vi "TGA_Configuration.vi"() -> ()   [LabVIEW 2016]
uses:
  TGA_Furnace_v230504.llb/LogInterval.ctl
  TGA_Furnace_v230504.llb/ChartWidth.ctl
  TGA_Furnace_v230504.llb/ADAM_models_enu.ctl
  TGA_Furnace_v230504.llb/Config_cluster.ctl
  TGA_Furnace_v230504.llb/HW_Config_cluster.ctl
  TGA_Furnace_v230504.llb/Adam_ID_cluster.ctl
  TGA_Furnace_v230504.llb/MFCs_ID_cluster.ctl
  TGA_Furnace_v230504.llb/MFC_ID_cluster.ctl
panel:
  in  "Gas Setpoints 3":T1={"Flow SP (l/min)"=15.0, "F1 N2 (%)"=79.99999999999997, "F1 H2 (%)"=0.0, "F1 CO (%)"=0.0, "F1 CO2 (%)"=20.00000000000003} caption="Gas Setpoints" {"F1 H2 (%)" min=0.0 max=100.0 step=0.1 format="%.1f"; "F1 CO2 (%)" min=0.0 max=100.0 step=0.1 format="%.1f"; "F1 CO (%)" min=0.0 max=100.0 step=0.1 format="%.1f"; "F1 N2 (%)" min=-10.0 max=100.0 format="%.1f"; "Flow SP (l/min)" min=0.0 max=30.0 format="%.1f"}
  in  "Gas Setpoints 2":T1={"Flow SP (l/min)"=15.0, "F1 N2 (%)"=79.99999999999997, "F1 H2 (%)"=0.0, "F1 CO (%)"=0.0, "F1 CO2 (%)"=20.00000000000003} caption="Gas Setpoints" {"F1 H2 (%)" min=0.0 max=100.0 step=0.1 format="%.1f"; "F1 CO2 (%)" min=0.0 max=100.0 step=0.1 format="%.1f"; "F1 CO (%)" min=0.0 max=100.0 step=0.1 format="%.1f"; "F1 N2 (%)" min=-10.0 max=100.0 format="%.1f"; "Flow SP (l/min)" min=0.0 max=30.0 format="%.1f"}
  in  "Gas Setpoints":T1={"Flow SP (l/min)"=15.0, "F1 N2 (%)"=79.99999999999997, "F1 H2 (%)"=0.0, "F1 CO (%)"=0.0, "F1 CO2 (%)"=20.00000000000003} {"F1 H2 (%)" min=0.0 max=100.0 step=0.1 format="%.1f"; "F1 CO2 (%)" min=0.0 max=100.0 step=0.1 format="%.1f"; "F1 CO (%)" min=0.0 max=100.0 step=0.1 format="%.1f"; "F1 N2 (%)" min=-10.0 max=100.0 format="%.1f"; "Flow SP (l/min)" min=0.0 max=30.0 format="%.1f"}
  out "Changed":bool
  in  "SaveAs_btn":bool
  in  "cancel_btn":bool
  in  "save_btn":bool
  in  "Tab Control":T2(tab)
  in  "Data directory path":path=path "C:/TGA/Data"
  in  "LogInterval":T3=1 items=["1 second"=1, "2 seconds"=2, "5 seconds"=5, "10 seconds"=10, "20 seconds"=20, "30 seconds"=30, "1 minute"=60, "2 minutes"=120, "5 minutes"=300]
  in  "LogStartComment":bool caption="Allow comment at start of logging."
  in  "LogEndComment":bool caption="Allow comment at end of logging"
  in  "GraphWidth":T4=1 items=["1 Minute", "5 Minutes", "10 Minutes", "30 Minutes", "1 Hour", "2 Hours"]
  in  "GraphSizeLimit":u16=7200
  in  "AlarmDelay":dbl=30.0 caption="N2 Flow Alarm\nDelay (s)"
  in  "Flow_error%":dbl=20.0 caption="N2 Low Flow\nError (%)"
  in  "TGA Gas File":string="Default" caption="Gas Filename"
  in  "Gas_SPs":T5={"Flow SP"=15.0, "N2 (%)"=70.0, "H2 (%)"=0.0, "CO (%)"=10.0, "CO2 (%)"=20.0} {"H2 (%)" min=0.0 max=100.0 format="%.1f"; "CO2 (%)" min=0.0 max=100.0 format="%.1f"; "CO (%)" min=0.0 max=100.0 format="%.1f"; "N2 (%)" min=-10.0 max=100.0 format="%.1f"; "Flow SP" min=0.0 max=30.0 format="%.1f"}
  out "ConfigFile path":path=path "C:/TGA/TGA_Main_v220630.cfg"
  out "MFCs_found":T6
  out "Adam_out_found":bool caption="Adam 4050"
  out "Euro_found":bool caption="Eurotherm"
  out "Balance_found":bool caption="Balance"
  in  "Adam_Out_ID":T8={"Serial Port"="COM7", "Model"=enum."4050", "Address"=1, "Slot"=0} caption="Adam Gas Solenoid\nOutput Module" {"Slot" max=7; "Address" min=1 max=254}
  in  "Euro_Address":u8=1 min=1 max=254
  in  "Euro_Port":refnum<visa-resource-name>="COM5" caption="Eurothem Temp.\nController Port"
  in  "Adam_In_ID":T8={"Serial Port"="COM6", "Model"=enum."4017", "Address"=2, "Slot"=0} caption="Adam Temp.\nInput Module" {"Slot" max=7; "Address" min=1 max=254}
  in  "Balance_Port":refnum<visa-resource-name>="COM4" caption="Radwag Balance\nSerial Port"
  in  "MFCs_Port":refnum<visa-resource-name>="COM10" caption="Brooks Mass Flow\nControllers Port"
  in  "test_btns":T9
  out "Adam_in_found":bool caption="Adam 4018"
  in  "MFC Device IDs":T10={"F1N2 MFC Device ID"={"MFC Device ID"=751101, "Type"=50}, "F1H2 MFC Device ID"={"MFC Device ID"=98201001, "Type"=100}, "F1CO MFC Device ID"={"MFC Device ID"=751201, "Type"=50}, "F1CO2 MFC Device ID"={"MFC Device ID"=98202001, "Type"=100}}
  # "TGA Configuration Editor"
  # "Type"
  # "Type"
  # "Type"
  # "Type"
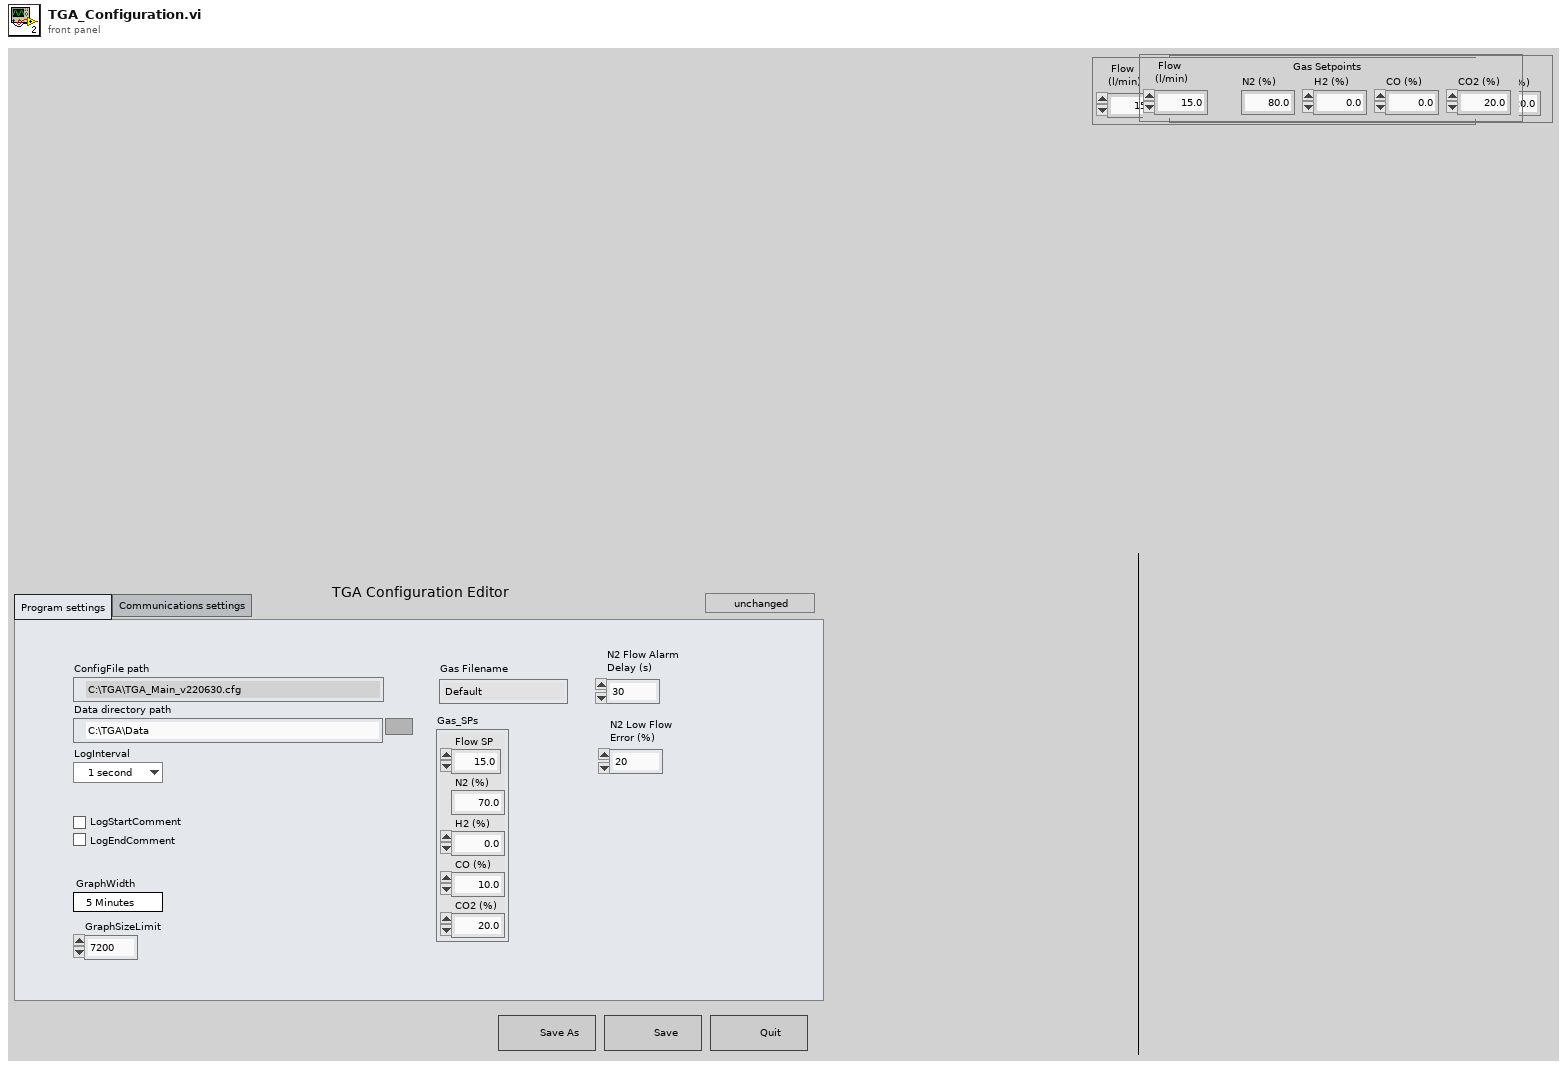
[diagram p1: front panel]
types:
  T1 = cluster{"Flow SP (l/min)":dbl, "F1 N2 (%)":dbl, "F1 H2 (%)":dbl, "F1 CO (%)":dbl, "F1 CO2 (%)":dbl}
  T2 = enum32{"Program settings", "Communications settings"}
  T3 = typedef "LogInterval.ctl" = u16
  T4 = typedef "ChartWidth.ctl" = u16
  T5 = cluster{"Flow SP":dbl, "N2 (%)":dbl, "H2 (%)":dbl, "CO (%)":dbl, "CO2 (%)":dbl}
  T6 = cluster{"Adam_out_found":bool, "Adam_out_found 2":bool, "Adam_out_found 3":bool, "Adam_out_found 4":bool}
  T7 = typedef "ADAM_models_enu.ctl" = enum16{"4011", "4012", "4013", "4015", "4015T", "4016", "4017", "4017+", "4018", "4018+", "4019+", "4019M", "4021", "4024", "4050", "4051", "4052", "4053", "4055", "4056S", "4056SO", "4060", "4068", "4069", "5000", "5017", "5018", "5024", "5051"}
  T8 = cluster{"Serial Port":refnum<visa-resource-name>, "Model":T7, "Address":u8, "Slot":u8}
  T9 = cluster{"test_bal_btn":bool, "test_adam_in":bool, "test_euro_btn":bool, "test_adam_out":bool, "test_MFCs_btn":bool}
  T10 = cluster{"F1N2 MFC Device ID":cluster{"MFC Device ID":u32, "Type":u8}, "F1H2 MFC Device ID":cluster{"MFC Device ID":u32, "Type":u8}, "F1CO MFC Device ID":cluster{"MFC Device ID":u32, "Type":u8}, "F1CO2 MFC Device ID":cluster{"MFC Device ID":u32, "Type":u8}}
  T11 = enum32{"Invalid", "Standard", "Closed", "Hidden", "Minimized", "Maximized"}
  T12 = typedef "Config_cluster.ctl" = cluster{"ConfigFile path":path, "Data directory path":path, "LogInterval":T3, "LogStartComment":bool, "LogEndComment":bool, "GraphWidth":T4, "GraphSizeLimit":u16, "HW_Config_cluster":T13, "TGA Gas File":string, "Gas_SPs":cluster{"Flow SP":dbl, "N2 (%)":dbl, "H2 (%)":dbl, "CO (%)":dbl, "CO2 (%)":dbl}, "AlarmDelay":dbl, "Flow_error%":dbl, "Purge Flow":dbl, "Gas_Times":cluster{"PrePurge Time":dbl, "Reduction Time":dbl, "Purge Time":dbl}, "Purge Setpoints":cluster{"F1 N2 (%)":dbl, "F1 H2 (%)":dbl, "F1 CO (%)":dbl, "F1 CO2 (%)":dbl}}
  T13 = typedef "HW_Config_cluster.ctl" = cluster{"Balance_Port":refnum<visa-resource-name>, "Adam_In_ID":T14, "Euro_Port":refnum<visa-resource-name>, "Euro_Address":u8, "Adam_Out_ID":T14, "MFCs_Port":refnum<visa-resource-name>, "MFC Device IDs":T15}
  T14 = typedef "Adam_ID_cluster.ctl" = cluster{"Serial Port":refnum<visa-resource-name>, "Model":T7, "Address":u8, "Slot":u8}
  T15 = typedef "MFCs_ID_cluster.ctl" = cluster{"F1N2 MFC Device ID":T16, "F1H2 MFC Device ID":T16, "F1CO MFC Device ID":T16, "F1CO2 MFC Device ID":T16}
  T16 = typedef "MFC_ID_cluster.ctl" = cluster{"MFC Device ID":u32, "Type":u8}
  T17 = cluster{"ConfigFile path":bool, "Data directory path":bool, "LogInterval":bool, "LogStartComment":bool, "LogEndComment":bool, "GraphWidth":bool, "GraphSizeLimit":bool, "HW_Config_cluster":cluster{"Balance_Port":bool, "Adam_In_ID":cluster{"Serial Port":bool, "Model":bool, "Address":bool, "Slot":bool}, "Euro_Port":bool, "Euro_Address":bool, "Adam_Out_ID":cluster{"Serial Port":bool, "Model":bool, "Address":bool, "Slot":bool}, "MFCs_Port":bool, "MFC Device IDs":cluster{"F1N2 MFC Device ID":cluster{"MFC Device ID":bool, "Type":bool}, "F1H2 MFC Device ID":cluster{"MFC Device ID":bool, "Type":bool}, "F1CO MFC Device ID":cluster{"MFC Device ID":bool, "Type":bool}, "F1CO2 MFC Device ID":cluster{"MFC Device ID":bool, "Type":bool}}}, "TGA Gas File":bool, "Gas_SPs":cluster{"Flow SP":bool, "N2 (%)":bool, "H2 (%)":bool, "CO (%)":bool, "CO2 (%)":bool}, "AlarmDelay":bool, "Flow_error%":bool, "Purge Flow":bool, "Gas_Times":cluster{"PrePurge Time":bool, "Reduction Time":bool, "Purge Time":bool}, "Purge Setpoints":cluster{"F1 N2 (%)":bool, "F1 H2 (%)":bool, "F1 CO (%)":bool, "F1 CO2 (%)":bool}}
  T18 = cluster{"Balance_Port":bool, "Adam_In_ID":cluster{"Serial Port":bool, "Model":bool, "Address":bool, "Slot":bool}, "Euro_Port":bool, "Euro_Address":bool, "Adam_Out_ID":cluster{"Serial Port":bool, "Model":bool, "Address":bool, "Slot":bool}, "MFCs_Port":bool, "MFC Device IDs":cluster{"F1N2 MFC Device ID":cluster{"MFC Device ID":bool, "Type":bool}, "F1H2 MFC Device ID":cluster{"MFC Device ID":bool, "Type":bool}, "F1CO MFC Device ID":cluster{"MFC Device ID":bool, "Type":bool}, "F1CO2 MFC Device ID":cluster{"MFC Device ID":bool, "Type":bool}}}
  T19 = cluster{"Flow SP":bool, "N2 (%)":bool, "H2 (%)":bool, "CO (%)":bool, "CO2 (%)":bool}
  T20 = cluster{"Serial Port":bool, "Model":bool, "Address":bool, "Slot":bool}
  T21 = cluster{"F1N2 MFC Device ID":cluster{"MFC Device ID":bool, "Type":bool}, "F1H2 MFC Device ID":cluster{"MFC Device ID":bool, "Type":bool}, "F1CO MFC Device ID":cluster{"MFC Device ID":bool, "Type":bool}, "F1CO2 MFC Device ID":cluster{"MFC Device ID":bool, "Type":bool}}
  T22 = cluster{"[0]":bool, "[1]":bool, "[2]":bool, "[3]":bool}
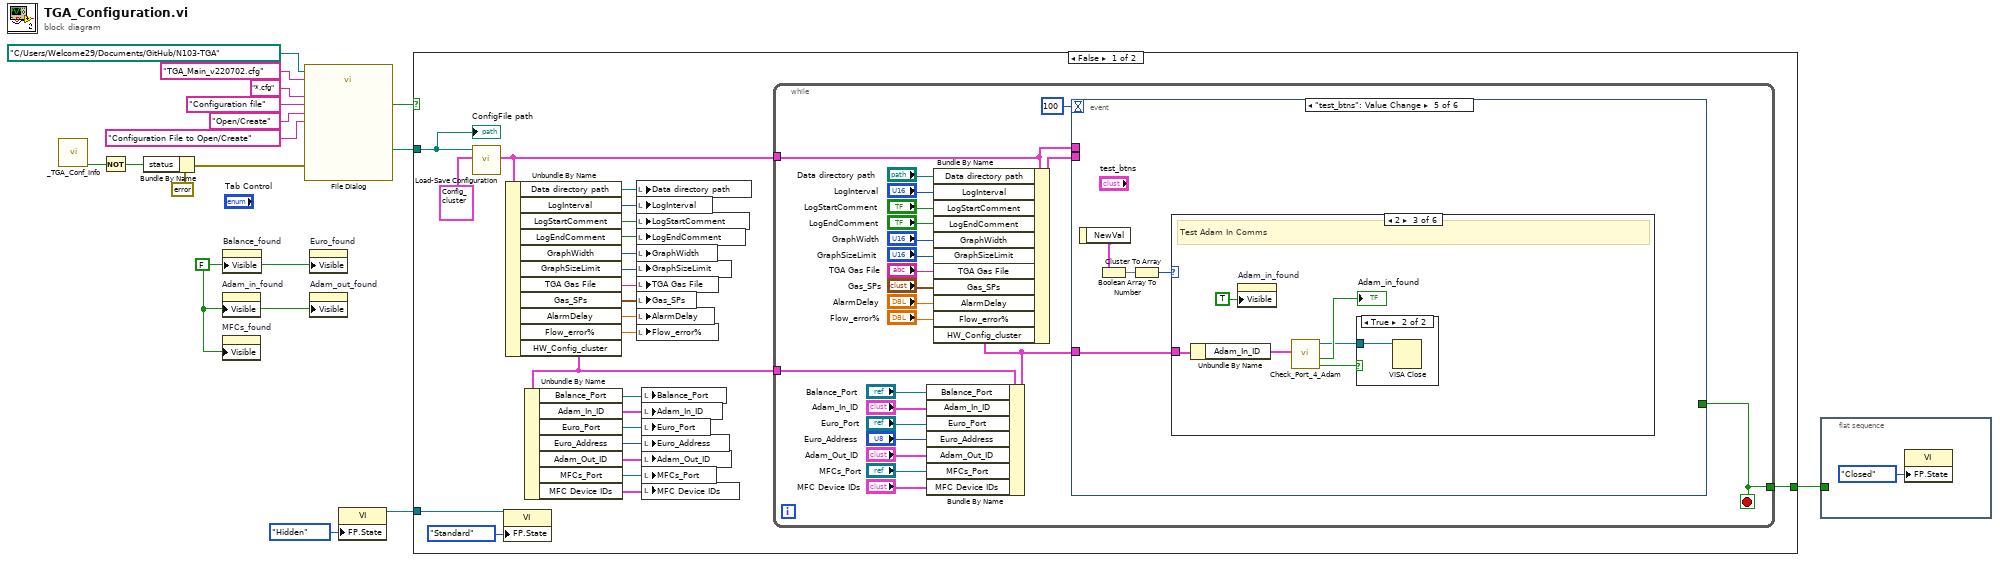
[diagram p0: block diagram]
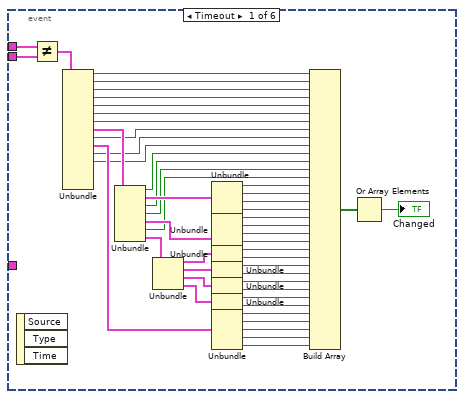
[diagram p2: hidden frame]
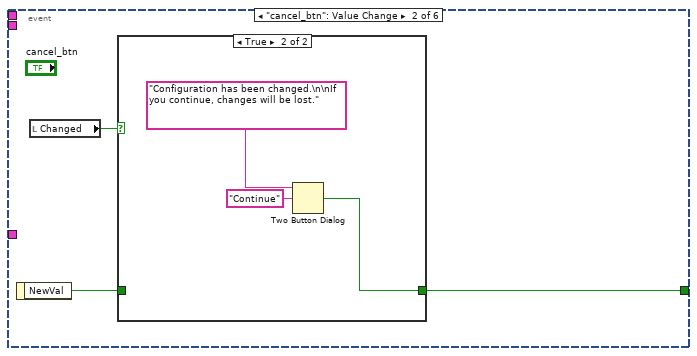
[diagram p3: hidden frame]
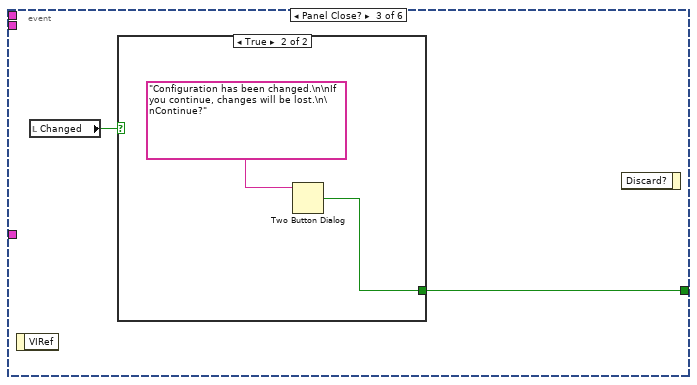
[diagram p5: hidden frame]
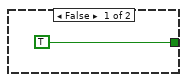
[diagram p6: hidden frame]
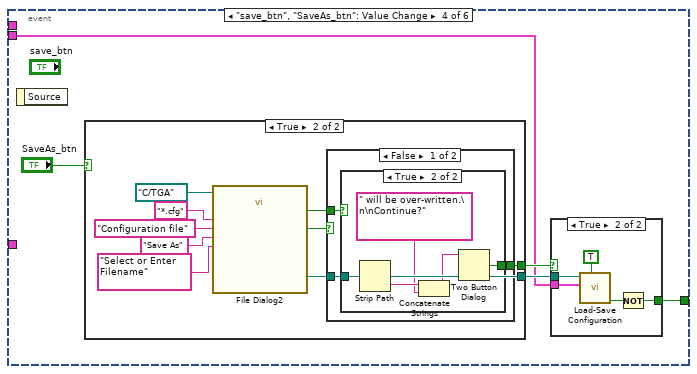
[diagram p7: hidden frame]
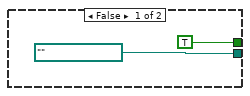
[diagram p9: hidden frame]
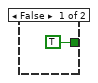
[diagram p10: hidden frame]
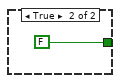
[diagram p11: hidden frame]
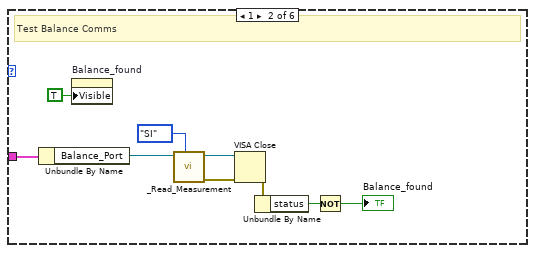
[diagram p13: hidden frame]
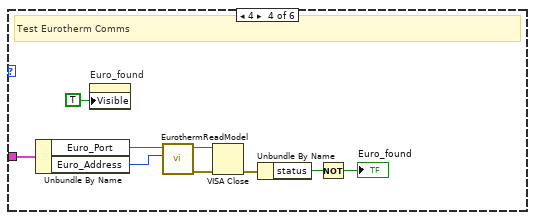
[diagram p15: hidden frame]
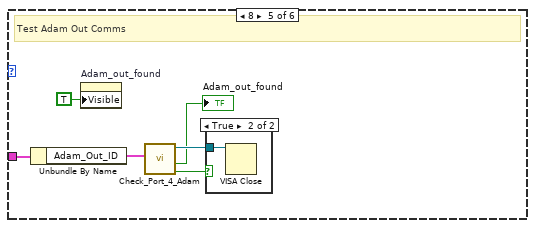
[diagram p16: hidden frame]
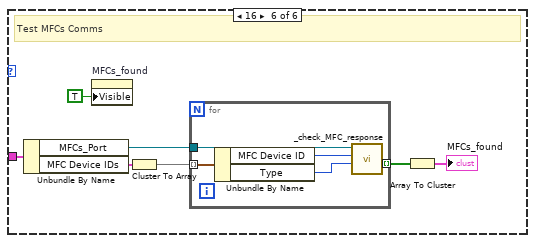
[diagram p18: hidden frame]
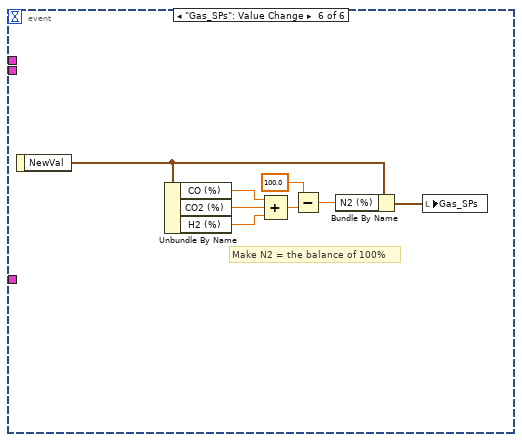
[diagram p19: hidden frame]
diagram:
  w9 = FALSE ("Visible")
  n1 = call "_TGA_Conf_Info.vi"() -> ("out"=w4:bool)  [unwired: 11 in]
  n2 = Not(x=w4) -> (.not. x?=w3:bool)
  n3 = Bundle By Name(cluster=errorcluster {"status"=FALSE, "code"=0, "source"=""} ("error in"), "status"=w3) -> (w5:errorcluster)
  n4 = property on="Adam_in_found" class="Bool (strict)"("Visible"=w9) -> ()  [unwired: 2 in, 2 out]
  n5 = property on="MFCs_found" class="Clust (strict)"("Visible"=w9) -> ()  [unwired: 2 in, 2 out]
  n6 = property on="Balance_found" class="Bool (strict)"("Visible"=w9) -> ()  [unwired: 2 in, 2 out]
  n7 = call "File Dialog"("start path"=path "C:/Users/Welcome29/Documents/GitHub/N103-TGA", "prompt"="Configuration File to Open/Create", "button label"="Open/Create", "default name"="TGA_Main_v220702.cfg", "error in"=w5, "pattern (all files)"="*.cfg", "pattern label"="Configuration file") -> ("selected path"=w10:path, "cancelled"=w11:bool)  [unwired: 5 in, 2 out]
  n8 = property on="Euro_found" class="Bool (strict)"("Visible"=w9) -> ()  [unwired: 2 in, 2 out]
  n9 = property on="Adam_out_found" class="Bool (strict)"("Visible"=w9) -> ()  [unwired: 2 in, 2 out]
  n10 = property class="VI"("FP.State"=T11."Hidden" ("Front Panel Window:State")) -> (reference out=w1:refnum<vi>)  [unwired: 2 in, 1 out]
  n11 = case shown="False" w11 {
    tunnel: w10 -> [w33 _]
    tunnel: [w19 _] -> w7
    tunnel: w1 -> [w17 _]
    frame False {
      n12 = call "Load-Save Configuration.vi"("Config Cluster"=T12 {"ConfigFile path"=path "", "Data directory path"=path "C:/TGA/Data", "LogInterval"=1, "LogStartComment"=FALSE, "LogEndComment"=FALSE, "GraphWidth"=1, "GraphSizeLimit"=7200, "HW_Config_cluster"={"Balance_Port"="COM4", "Adam_In_ID"={"Serial Port"="COM6", "Model"=enum."4017", "Address"=1, "Slot"=0}, "Euro_Port"="COM5", "Euro_Address"=1, "Adam_Out_ID"={"Serial Port"="COM7", "Model"=enum."4050", "Address"=1, "Slot"=0}, "MFCs_Port"="COM10", "MFC Device IDs"={"F1N2 MFC Device ID"={"MFC Device ID"=751101, "Type"=50}, "F1H2 MFC Device ID"={"MFC Device ID"=201001, "Type"=100}, "F1CO MFC Device ID"={"MFC Device ID"=751201, "Type"=50}, "F1CO2 MFC Device ID"={"MFC Device ID"=202001, "Type"=100}}}, "TGA Gas File"="Defalt_Gasfile", "Gas_SPs"={"Flow SP"=15.0, "N2 (%)"=70.0, "H2 (%)"=0.0, "CO (%)"=10.0, "CO2 (%)"=20.0}, "AlarmDelay"=30.0, "Flow_error%"=20.0, "Purge Flow"=0.0, "Gas_Times"={"PrePurge Time"=0.0, "Reduction Time"=0.0, "Purge Time"=0.0}, "Purge Setpoints"={"F1 N2 (%)"=99.0, "F1 H2 (%)"=1.0, "F1 CO (%)"=0.0, "F1 CO2 (%)"=0.0}}, "ConfigFile path (Not A Path)"=w33) -> ("Config Cluster out"=w32:T12)  [unwired: 6 in, 1 out]
      n13 = property class="VI"(reference=w17, "FP.State"=T11."Standard" ("Front Panel Window:State")) -> ()  [unwired: 1 in, 2 out]
      n14 = Unbundle By Name(w32) -> ("Data directory path"=w22:path, "LogInterval"=w23:T3, "LogStartComment"=w24:bool, "LogEndComment"=w25:bool, "GraphWidth"=w26:T4, "GraphSizeLimit"=w27:u16, "TGA Gas File"=w28:string, "Gas_SPs"=w29:T5, "AlarmDelay"=w30:dbl, "Flow_error%"=w31:dbl, "HW_Config_cluster"=w21:T13)
      n15 = Unbundle By Name(w21) -> ("Balance_Port"=w40:refnum<visa-resource-name>, "Adam_In_ID"=w39:T14, "Euro_Port"=w38:refnum<visa-resource-name>, "Euro_Address"=w37:u8, "Adam_Out_ID"=w36:T14, "MFCs_Port"=w35:refnum<visa-resource-name>, "MFC Device IDs"=w34:T15)
      n16 = local write "Data directory path"(w22) -> ()
      n17 = local write "LogInterval"(w23) -> ()
      n18 = local write "LogStartComment"(w24) -> ()
      n19 = local write "LogEndComment"(w25) -> ()
      n20 = local write "GraphWidth"(w26) -> ()
      n21 = local write "GraphSizeLimit"(w27) -> ()
      n22 = local write "TGA Gas File"(w28) -> ()
      n23 = local write "Gas_SPs"(w29) -> ()
      n24 = local write "AlarmDelay"(w30) -> ()
      n25 = local write "Flow_error%"(w31) -> ()
      n26 = local write "Balance_Port"(w40) -> ()
      n27 = local write "Adam_In_ID"(w39) -> ()
      n28 = local write "Euro_Port"(w38) -> ()
      n29 = local write "Euro_Address"(w37) -> ()
      n30 = local write "Adam_Out_ID"(w36) -> ()
      n31 = local write "MFCs_Port"(w35) -> ()
      n32 = local write "MFC Device IDs"(w34) -> ()
      n33 = while {
        tunnel: w32 -> [w43]
        tunnel: w21 -> [w45]
        tunnel: [w41] -> w19
        stop <- w41 stop-if-true
        n34 = Bundle By Name(cluster=w45, "Balance_Port"="Balance_Port", "Adam_In_ID"="Adam_In_ID", "Euro_Port"="Euro_Port", "Euro_Address"="Euro_Address", "Adam_Out_ID"="Adam_Out_ID", "MFCs_Port"="MFCs_Port", "MFC Device IDs"="MFC Device IDs") -> (w42:T13)
        n35 = Bundle By Name(cluster=w43, "Data directory path"="Data directory path", "LogInterval"="LogInterval", "LogStartComment"="LogStartComment", "LogEndComment"="LogEndComment", "GraphWidth"="GraphWidth", "GraphSizeLimit"="GraphSizeLimit", "TGA Gas File"="TGA Gas File", "Gas_SPs"="Gas_SPs", "AlarmDelay"="AlarmDelay", "Flow_error%"="Flow_error%", "HW_Config_cluster"=w42) -> (w53:T12)
        n36 = event shown="[4] \"test_btns\": Value Change" {
          selector: _ -> [_ _ _ _ _ _]
          dyn-events: _ -> [_ _ _ _ _ _]
          timeout: 100 -> [_ _ _ _ _ _]
          tunnel: [_ w114 w120 w126 _ _] -> w41
          tunnel: w53 -> [w111 _ _ w125 _ _]
          tunnel: w43 -> [w112 _ _ _ _ _]
          tunnel: w42 -> [_ _ _ _ w157 _]
          event Timeout {
            n37 = event-data() -> ()  [unwired: 1 in, 3 out]
            n38 = Not Equal?(x=w112, y=w111) -> (x != y?=w110:T17)
            n39 = Unbundle(w110) -> ("ConfigFile path"=w104:bool, "Data directory path"=w103:bool, "LogInterval"=w102:bool, "LogStartComment"=w101:bool, "LogEndComment"=w100:bool, "GraphWidth"=w99:bool, "GraphSizeLimit"=w98:bool, "HW_Config_cluster"=w109:T18, "TGA Gas File"=w97:bool, "Gas_SPs"=w105:T19, "AlarmDelay"=w96:bool, "Flow_error%"=w95:bool)  [unwired: 3 out]
            n40 = Unbundle(w109) -> ("Balance_Port"=w94:bool, "Adam_In_ID"=w108:T20, "Euro_Port"=w93:bool, "Euro_Address"=w92:bool, "Adam_Out_ID"=w107:T20, "MFCs_Port"=w91:bool, "MFC Device IDs"=w106:T21)
            n41 = Unbundle(w106) -> ("F1N2 MFC Device ID"=w75:cluster{"MFC Device ID":bool, "Type":bool}, "F1H2 MFC Device ID"=w70:cluster{"MFC Device ID":bool, "Type":bool}, "F1CO MFC Device ID"=w72:cluster{"MFC Device ID":bool, "Type":bool}, "F1CO2 MFC Device ID"=w71:cluster{"MFC Device ID":bool, "Type":bool})
            n42 = Unbundle(w108) -> ("Serial Port"=w90:bool, "Model"=w89:bool, "Address"=w88:bool, "Slot"=w87:bool)
            n43 = Unbundle(w107) -> ("Serial Port"=w86:bool, "Model"=w85:bool, "Address"=w84:bool, "Slot"=w83:bool)
            n44 = Unbundle(w75) -> ("MFC Device ID"=w74:bool, "Type"=w73:bool)
            n45 = Unbundle(w70) -> ("MFC Device ID"=w69:bool, "Type"=w68:bool)
            n46 = Unbundle(w72) -> ("MFC Device ID"=w67:bool, "Type"=w66:bool)
            n47 = Unbundle(w71) -> ("MFC Device ID"=w65:bool, "Type"=w64:bool)
            n48 = Unbundle(w105) -> ("Flow SP"=w82:bool, "N2 (%)"=w81:bool, "H2 (%)"=w80:bool, "CO (%)"=w79:bool, "CO2 (%)"=w78:bool)
            n49 = Build Array(w104, w103, w102, w101, w100, w99, w98, w97, w96, w95, w94, w93, w92, w91, w90, w89, w88, w87, w86, w85, w84, w83, w74, w73, w69, w68, w67, w66, w65, w64, w82, w81, w80, w79, w78) -> (w77:bool[])
            n50 = Or Array Elements(Boolean array=w77) -> (logical OR=→"Changed":bool)
          }
          event "cancel_btn": Value Change {
            n51 = event-data() -> ("NewVal"=w113:bool)  [unwired: 1 in]
            n52 = local read "Changed"() -> (w115:bool)
            n53 = case shown="True" w115 {
              tunnel: [w116 w118] -> w114
              tunnel: w113 -> [w116 _]
              frame False {
              }
              frame True {
                n54 = Two Button Dialog(message="Configuration has been changed.\n\nIf you continue, changes will be lost.", 2:"Continue" ("T button name (\"OK\")")) -> (T button?=w118:bool)  [unwired: 1 in]
              }
            }
          }
          event Panel Close? {
            n55 = event-data() -> ()  [unwired: 1 in, 1 out]
            n56 = local read "Changed"() -> (w121:bool)
            n57 = case shown="True" w121 {
              tunnel: [TRUE ("T button?") w123] -> w120
              frame False {
              }
              frame True {
                n58 = Two Button Dialog(message="Configuration has been changed.\n\nIf you continue, changes will be lost.\n\nContinue?") -> (T button?=w123:bool)  [unwired: 2 in]
              }
            }
            n59 = event-data() -> ()  [unwired: 2 in, 1 out]
          }
          event "save_btn", "SaveAs_btn": Value Change {
            n60 = event-data() -> ()  [unwired: 1 in, 1 out]
            n61 = case shown="True" "SaveAs_btn" {
              tunnel: [TRUE ("T button?") w139] -> w128
              tunnel: [path "" ("selected path") w138] -> w127
              frame False {
              }
              frame True {
                n62 = call "File Dialog2"("start path"=path "C:/TGA", "prompt"="Select or Enter Filename", "button label"="Save As", "pattern (all files)"="*.cfg", "pattern label"="Configuration file") -> ("selected path"=w138:path, "exists"=w140:bool, "cancelled"=w141:bool)  [unwired: 7 in, 1 out]
                n63 = case shown="False" w141 {
                  tunnel: w140 -> [w149 _]
                  tunnel: w138 -> [w148 _]
                  tunnel: [w147 FALSE] -> w139
                  frame False {
                    n64 = case shown="True" w149 {
                      tunnel: w148 -> [_ w155]
                      tunnel: [TRUE w151] -> w147
                      frame False {
                      }
                      frame True {
                        n65 = Strip Path(path=w155) -> (name=w154:string)  [unwired: 1 out]
                        n66 = Concatenate Strings(w154, " will be over-written.\n\nContinue?" ("message")) -> (w152:string)
                        n67 = Two Button Dialog(message=w152) -> (T button?=w151:bool)  [unwired: 2 in]
                      }
                    }
                  }
                  frame True {
                  }
                }
              }
            }
            n68 = case shown="True" w128 {
              selector: w128 -> [w130 _]
              tunnel: w125 -> [_ w134]
              tunnel: w127 -> [_ w133]
              tunnel: [w130 w131] -> w126
              frame False {
              }
              frame True {
                n69 = call "Load-Save Configuration.vi"("Save (F: Load)"=TRUE, "Config Cluster"=w134, "ConfigFile path (Not A Path)"=w133) -> ("Error"=w132:bool)  [unwired: 5 in, 1 out]
                n70 = Not(x=w132) -> (.not. x?=w131:bool)
              }
            }
          }
          event "test_btns": Value Change {
            n71 = event-data() -> ("NewVal"=w160:T9)  [unwired: 1 in]
            n72 = Cluster To Array(cluster=w160) -> (array=w159:bool[])
            n73 = Boolean Array To Number(Boolean array=w159) -> (number=w158:u32)
            n74 = case shown="2" w158 {
              tunnel: w157 -> [_ w167 w174 w183 w190 w199]
              frame 0, Default {
              }
              frame 1 {
                # "Test Balance Comms"
                n75 = Unbundle By Name(w167) -> ("Balance_Port"=w166:refnum<visa-resource-name>)
                n76 = property on="Balance_found" class="Bool (strict)"("Visible"=TRUE) -> ()  [unwired: 2 in, 2 out]
                n77 = call "_Read_Measurement.vi"("Cmd"=enum16{"S", "SI", "SU", "SUI"}."SI", "VISA resource name"=w166) -> ("error out"=w165:errorcluster, "VISA resource out"=w169:refnum<visa-resource-name>)  [unwired: 6 in, 2 out]
                n78 = VISA Close(VISA resource name=w169, error in (no error)=w165) -> (error out=w164:errorcluster)
                n79 = Unbundle By Name(w164) -> ("status"=w163:bool)
                n80 = Not(x=w163) -> (.not. x?=→"Balance_found":bool)
              }
              frame 2 {
                # "Test Adam In Comms"
                n81 = Unbundle By Name(w174) -> ("Adam_In_ID"=w173:T14)
                n82 = property on="Adam_in_found" class="Bool (strict)"("Visible"=TRUE) -> ()  [unwired: 2 in, 2 out]
                n83 = call "Check_Port_4_Adam.vi"("Adam_ID_cluster"=w173) -> ("Port Opened"=w170:bool, "Found"=→"Adam_in_found":bool, "VISA name out"=w171:refnum<visa-resource-name>)  [unwired: 6 in, 2 out]
                n84 = case shown="True" w170 {
                  tunnel: w171 -> [_ w176]
                  frame False {
                  }
                  frame True {
                    n85 = VISA Close(VISA resource name=w176) -> ()  [unwired: 1 in, 1 out]
                  }
                }
              }
              frame 4 {
                # "Test Eurotherm Comms"
                n86 = Unbundle By Name(w183) -> ("Euro_Port"=w182:refnum<visa-resource-name>, "Euro_Address"=w181:u8)
                n87 = property on="Euro_found" class="Bool (strict)"("Visible"=TRUE) -> ()  [unwired: 2 in, 2 out]
                n88 = call "EurothermReadModel.vi"("Device Address (1)"=w181, "VISA name"=w182) -> ("error out"=w184:errorcluster, "VISA name out"=w185:refnum<visa-resource-name>)  [unwired: 6 in, 2 out]
                n89 = VISA Close(VISA resource name=w185, error in (no error)=w184) -> (error out=w180:errorcluster)
                n90 = Unbundle By Name(w180) -> ("status"=w179:bool)
                n91 = Not(x=w179) -> (.not. x?=→"Euro_found":bool)
              }
              frame 8 {
                # "Test Adam Out Comms"
                n92 = Unbundle By Name(w190) -> ("Adam_Out_ID"=w189:T14)
                n93 = property on="Adam_out_found" class="Bool (strict)"("Visible"=TRUE) -> ()  [unwired: 2 in, 2 out]
                n94 = call "Check_Port_4_Adam.vi"("Adam_ID_cluster"=w189) -> ("Port Opened"=w186:bool, "Found"=→"Adam_out_found":bool, "VISA name out"=w188:refnum<visa-resource-name>)  [unwired: 6 in, 2 out]
                n95 = case shown="True" w186 {
                  tunnel: w188 -> [_ w192]
                  frame False {
                  }
                  frame True {
                    n96 = VISA Close(VISA resource name=w192) -> ()  [unwired: 1 in, 1 out]
                  }
                }
              }
              frame 16 {
                # "Test MFCs Comms"
                n97 = Unbundle By Name(w199) -> ("MFCs_Port"=w198:refnum<visa-resource-name>, "MFC Device IDs"=w197:T15)
                n98 = property on="MFCs_found" class="Clust (strict)"("Visible"=TRUE) -> ()  [unwired: 2 in, 2 out]
                n99 = Cluster To Array(cluster=w197) -> (array=w196:T16[])
                n100 = for {
                  tunnel: w198 -> [w204]
                  tunnel: w196 -> [w202] mode=indexing
                  tunnel: [w203] -> w194 mode=indexing
                  n101 = Unbundle By Name(w202) -> ("MFC Device ID"=w201:u32, "Type"=w200:u8)
                  n102 = call "_check_MFC_response.vi"("Device Type"=w200, "Device ID"=w201, "MFCs_Port"=w204) -> ("Found"=w203:bool)  [unwired: 4 in, 2 out]
                }
                n103 = Array To Cluster(array=w194) -> (cluster=→"MFCs_found":T22)
              }
            }
          }
          event "Gas_SPs": Value Change {
            (unwired) 100.0 ("y")
            (unwired) 100.0 ("y")
            (unwired) 100.0 ("y")
            # "Make N2 = the balance of 100%"
            # "Make N2 = the balance of 100%"
            # "Make N2 = the balance of 100%"
            # "Make N2 = the balance of 100%"
            n104 = event-data() -> ("NewVal"=w205:T5)  [unwired: 1 in]
            n105 = Unbundle By Name(w205) -> ("CO (%)"=w211:dbl, "CO2 (%)"=w210:dbl, "H2 (%)"=w209:dbl)
            n106 = Compound Arithmetic op=ADD(w211, w210, w209) -> (w207:dbl)
            n107 = Subtract(x=100.0 ("y"), y=w207) -> (x-y=w206:dbl)
            n108 = Bundle By Name(cluster=w205, "N2 (%)"=w206) -> (w212:T5)
            n109 = local write "Gas_SPs"(w212) -> ()
          }
        }
      }
      "ConfigFile path" <- w33
    }
    frame True {
    }
  }
  n110 = flat-sequence {
    tunnel: w7 -> [_]
    frame #0 {
      n111 = property class="VI"("FP.State"=T11."Closed" ("Front Panel Window:State")) -> ()  [unwired: 2 in, 2 out]
    }
  }
